vi "myRIO_BRig_Host_test_dataGeneration_main.vi"(10 "nTrial_perBlock":u16, 11 "nTrial_total":u16) -> (2 "output_streamData":u16[][](array[numeric]), 3 "output_fileData":u16[][](array[numeric]))   [LabVIEW 2014]
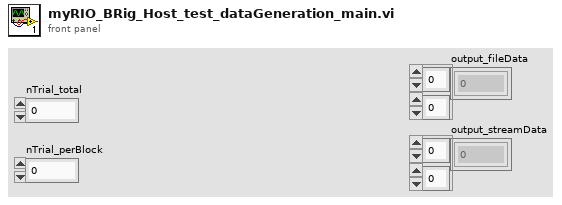
[diagram p1: front panel]
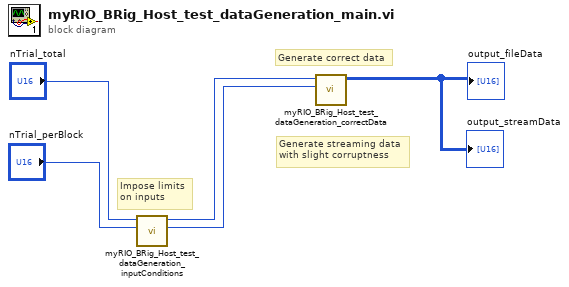
[diagram p0: block diagram]
diagram:
  # "Generate streaming data\nwith slight corruptness"
  # "Impose limits\non inputs"
  # "Generate correct data"
  n1 = call "myRIO_BRig_Host_test_dataGeneration_inputConditions.vi"("nTrial_perBlock"="nTrial_perBlock", "input_nTrial_total"="nTrial_total") -> ("output_nTrial_perBlock"=w2:u16, "output_nTrial_total"=w3:u16)  [unwired: 8 in]
  n2 = call "myRIO_BRig_Host_test_dataGeneration_correctData.vi"("input_nTrial_perBlock"=w2, "input_nTrial_total"=w3) -> ("output_correctData"=→"output_fileData" →"output_streamData":u16[][])  [unwired: 9 in]
